vi "Read Status Source.vi"(8 "error in (no error)":errorcluster, 11 "Session in":refnum<class "Session.lvclass">) -> (0 "error out":errorcluster, 2 "Status Source":T1, 3 "Session out":refnum<class "Session.lvclass">)   [LabVIEW 2024, in "CTI.lvlib" / "Session.lvclass"]
doc: "Returns the current configuration that determines when the status LED for a device lights up. See <b>Write Status Source.vi</b> for a description of the available status sources."
uses:
  Session.lvclass
  Status Source.ctl
  DeviceComms/DeviceComms.lvclass
  CTI.lvlib
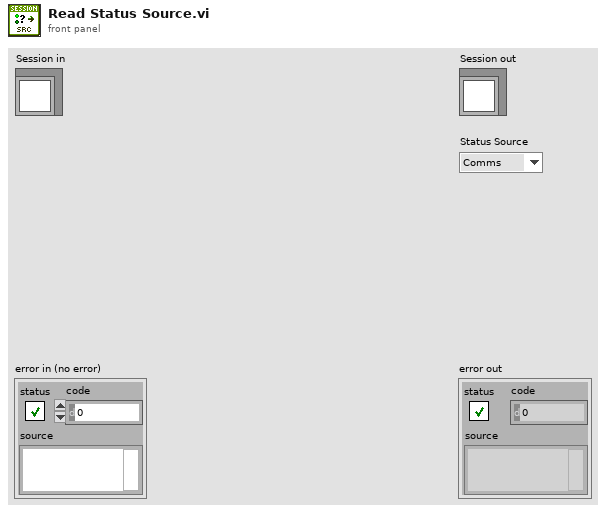
[diagram p1: front panel]
types:
  T1 = typedef "CTI.lvlib/Status Source.ctl" = enum16{"Comms", "User"}
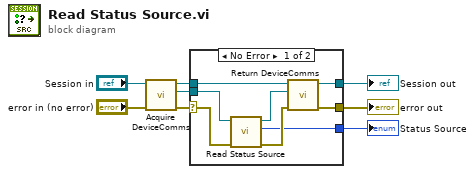
[diagram p0: block diagram]
diagram:
  n1 = call "Acquire DeviceComms.vi"("error in (no error)"="error in (no error)", "Session in"="Session in") -> ("error out"=w4:errorcluster, "DeviceComms"=w5:refnum<class "DeviceComms.lvclass">, "Session out"=w6:refnum<class "Session.lvclass">)  [unwired: 7 in]
  n2 = case shown="No Error" w4 {
    selector: w4 -> [w14 w17]
    tunnel: w6 -> [w16 w18]
    tunnel: w5 -> [w15 _]
    tunnel: [w13 w18] -> w3
    tunnel: [w10 _] -> w2
    tunnel: [w9 w17] -> w1
    frame No Error {
      n3 = call-dynamic "Read Status Source.vi"("error in (no error)"=w14, "DeviceComms in"=w15) -> ("error out"=w11:errorcluster, "Status Source"=w10:T1, "DeviceComms out"=w12:refnum<class "DeviceComms.lvclass">)  [unwired: 7 in]
      n4 = call "Return DeviceComms.vi"("error in (no error)"=w11, "DeviceComms"=w12, "Session in"=w16) -> ("error out"=w9:errorcluster, "Session out"=w13:refnum<class "Session.lvclass">)  [unwired: 7 in]
    }
    frame Error {
    }
  }
  "error out" <- w1
  "Session out" <- w3
  "Status Source" <- w2
